vi "Parse FRC TimeStamp String.vi"(11 "date/time string":string) -> (2 "year":i32, 3 "Resulting Time Stamp":timestamp)   [LabVIEW 2014, in "FIRST Events API.lvlib"]
uses:
  FIRST Events API.lvlib
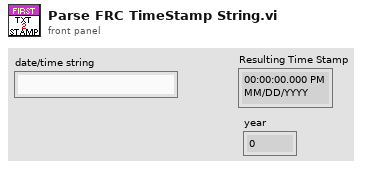
[diagram p1: front panel]
types:
  T1 = cluster{"second":i32, "minute":i32, "hour":i32, "day of month":i32, "month":i32, "year":i32, "day of week":i32, "day of year":i32, "is DST":i32}
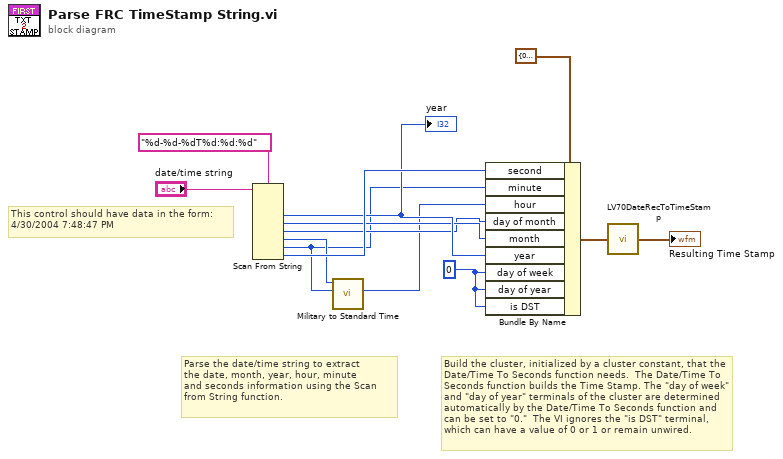
[diagram p0: block diagram]
diagram:
  w8 = 0
  # "This control should have data in the form:\n4/30/2004 7:48:47 PM"
  # "Build the cluster, initialized by a cluster constant, that the Date/Time To Seconds function needs.  The Date/Time To Seconds function builds the Time Stamp. The \"day of week\" and \"day of year\" terminals of the cluster are determined automatically by the Date/Time To Seconds function and can be set to \"0.\"  The VI ignores the \"is DST\" terminal, which can have a value of 0 or 1 or remain unwired."
  # "Parse the date/time string to extract \nthe date, month, year, hour, minute \nand seconds information using the Scan\nfrom String function."
  n1 = Scan From String "Scan From String"(format string="%d-%d-%dT%d:%d:%d", input string="date/time string") -> (output 1=w6:i32, output 2=w5:i32, output 3=w4:i32, output 4=w3:i32, output 5=w2:i32, output 6=w7:i32)  [unwired: 8 in, 3 out]
  "year" <- w6
  n2 = call "Military to Standard Time.vi"("Minute"=w2, "Hour"=w3) -> ("Hour"=w1:i32)  [unwired: 7 in, 2 out]
  n3 = Bundle By Name(cluster=T1 {"second"=0, "minute"=0, "hour"=0, "day of month"=0, "month"=0, "year"=0, "day of week"=0, "day of year"=0, "is DST"=0} ("date time rec"), "second"=w7, "minute"=w2, "hour"=w1, "day of month"=w4, "month"=w5, "year"=w6, "day of week"=w8, "day of year"=w8, "is DST"=w8) -> (w9:T1)
  n4 = call <vilib>:"LV70DateRecToTimeStamp.vi"("date time rec"=w9) -> ("Time Stamp"=→"Resulting Time Stamp":timestamp)
